vi "CRC.vi"(0 "object in":refnum<class "212format_work.lvclass">, 1 "puchMsg":string, 5 "error in (no error)":errorcluster) -> (14 "object out":refnum<class "212format_work.lvclass">, 15 "数据段长度":string, 16 "数据段":string, 17 "CRC校验":string, 19 "error out":errorcluster)   [LabVIEW 2016]
uses:
  212format_work.lvclass
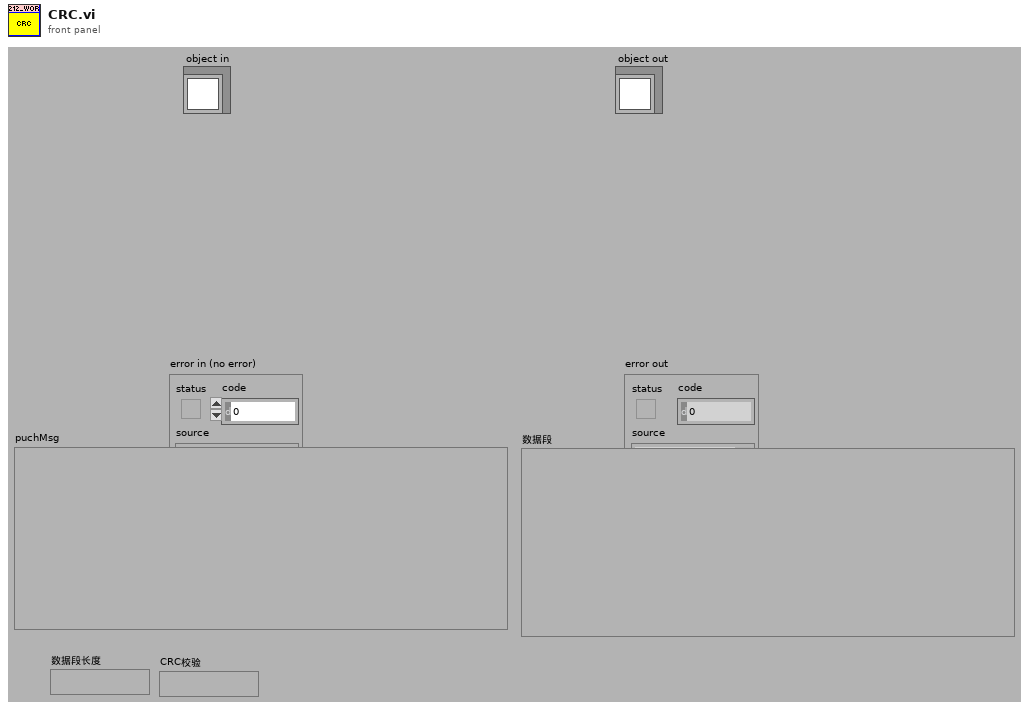
[diagram p1: front panel]
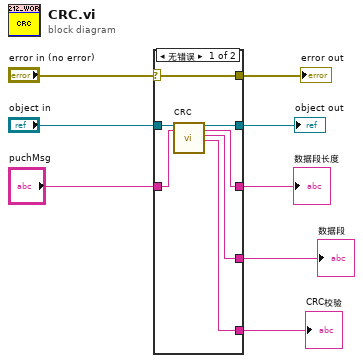
[diagram p0: block diagram]
diagram:
  n1 = case shown="无错误" "error in (no error)" {
    selector: "error in (no error)" -> [w15 w17]
    tunnel: [w15 w17] -> w7
    tunnel: [w11 w16] -> w5
    tunnel: "object in" -> [w12 w16]
    tunnel: [w14 _] -> w4
    tunnel: "puchMsg" -> [w13 _]
    tunnel: [w10 _] -> w2
    tunnel: [w9 _] -> w1
    frame No Error {
      n2 = call-dynamic "CRC.vi"("object in"=w12, "puchMsg"=w13) -> ("object out"=w11:refnum<class "212format_work.lvclass">, "数据段长度"=w9:string, "数据段"=w10:string, "CRC校验"=w14:string)  [unwired: 13 in, 1 out]
    }
    frame Error {
    }
  }
  "error out" <- w7
  "object out" <- w5
  "数据段长度" <- w1
  "数据段" <- w2
  "CRC校验" <- w4
